vi "Parse Parameters.vi"(10 "String":string, 11 "Array in":dbl[](array[numeric])) -> (3 "Array out":dbl[](array[numeric]))   [LabVIEW 2024]
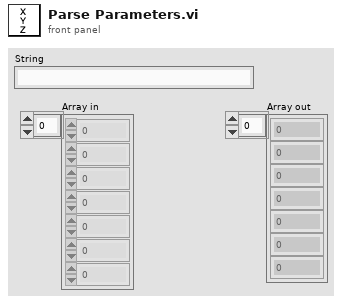
[diagram p1: front panel]
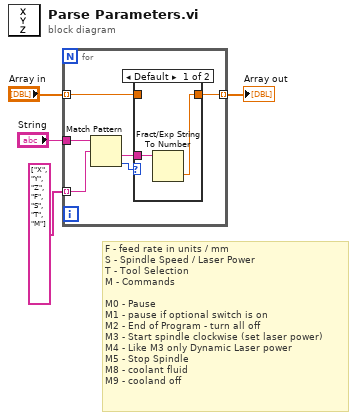
[diagram p0: block diagram]
diagram:
  # "F - feed rate in units / mm\nS - Spindle Speed / Laser Power\nT - Tool Selection\nM - Commands\n\nM0 - Pause\nM1 - pause if optional switch is on\nM2 - End of Program - turn all off\nM3 - Start spindle clockwise (set laser power)\nM4 - Like M3 only Dynamic Laser power\nM5 - Stop Spindle\nM8 - coolant fluid\nM9 - cooland off"
  n1 = for {
    tunnel: string[] ["X", "Y", "Z", "F", "S", "T", "M"] -> [w10] mode=indexing
    tunnel: "String" -> [w9]
    tunnel: [w6] -> w2 mode=indexing
    tunnel: "Array in" -> [w5] mode=indexing
    n2 = Match Pattern(string=w9, regular expression=w10) -> (after substring=w7:string, offset past match=w8:i32)  [unwired: 1 in, 2 out]
    n3 = case shown="Default" w8 {
      tunnel: w7 -> [w12 _]
      tunnel: [w11 w13] -> w6
      tunnel: w5 -> [_ w13]
      frame Default {
        n4 = Fract/Exp String To Number(string=w12) -> (number=w11:dbl)  [unwired: 3 in, 1 out]
      }
      frame -1 {
      }
    }
  }
  "Array out" <- w2
